vi "PhysioMoment.vi"() -> ()   [LabVIEW 2012]
doc: "Demonstrates general use of Obtain Queue, queues and the effects different settings have on queue behavior. It uses a queue to pass data between an Enqueue loop (producing data) and a Dequeue loop (consuming data). If both loops run at the same speed, the queue does not fill up.\n\nWhen the Enqueue loop runs fast and the Dequeue loop runs slow, the queue quickly fills up and the Enqueue loop must wait for the Dequeue loop to remove elements. If the Enqueue loop runs slow and the Dequeue loop runs fast, the queue is quickly emptied and the Dequeue loop must wait for the Enqueue loop to insert elements."
uses:
  <vilib>/Utility/file.llb/Read From Spreadsheet File (DBL).vi
  global_variable/tvi_arx_ni9234_global.vi
  <vilib>/Utility/file.llb/Read From Spreadsheet File (I64).vi
  <vilib>/Analysis/baseanly.llb/Mean (DBL).vi
  <vilib>/Analysis/NI_AALBase.lvlib
  <vilib>/Analysis/NI_AALPro.lvlib
panel:
  out "String":string="Ground Reaction Force \nBio-FeedBack System"
  out "output data size 2":i32
  out "transfer data size":i32
  out "transfer data":csg[](array[numeric])
  in  "Tab Control 2":enum32{"Settings", "Main Panel"}(tab)
  in  "Hours":i32
  in  "minutes":i32=14
  in  "seconds":i32
  in  "Loadcell Output Data":path
  in  "Led Runner File":path
  in  "Led Text File":path
  in  "Transfer Function":path
  out "Hours":i32
  out "minutes  2":i32=30
  out "seconds":i32
  in  "stop":bool
  in  "Tab Control":enum32{"GRF", "Raw Data"}(tab)
  out "10 SLOPE INCREMENT":dbl format="%#_3g"
  out "10 STRIDE INCREMENT":dbl format="%#_3g"
  out "5 SLOPE INCREMENT":dbl format="%#_3g"
  out "5 STRIDE INCREMENT":dbl format="%#_3g"
  out "1 SLOPE INCREMENT":dbl format="%#_3g"
  out "1 STRIDE INCREMENT":dbl format="%#_3g"
  out "TVItv SCORE":dbl format="%#_3g"
  out "Slope SCORE":dbl format="%#_3g"
  out "TVItv SCORE":dbl format="%#_3g"
  out "Slope SCORE":dbl format="%#_3g"
  out "Slope SCORE":dbl format="%#_3g"
  out "TVItv SCORE":dbl format="%#_3g"
  out "Bio-Feedback System":bool[][](array[boolean])
  out "Right Foot GRF":cluster{dbl[], "Z-Score":dbl[]}[](graph)
  out "Left Foot GRF":cluster{dbl[], "Z-Score":dbl[]}[](graph)
  out "TVItv Score : 1 stride":cluster{i32[], "Best Linear Fit":dbl[]}[](graph)
  out "TVItv Score : 5 strides":cluster{i32[], "Best Linear Fit":dbl[]}[](graph)
  out "TVItv Score : 10 strides":cluster{i32[], "Best Linear Fit":dbl[]}[](graph)
  out "GRF Output":dbl[](graph)
  out "GRF Input Waveform (2 Second Window)":cluster{dbl[], "Z-Score":dbl[]}[](graph)
  out "Step Interval (sec)":dbl
  out "tvit pr (1 strides)":dbl
  out "led loop execute time":dbl
  out "tvit (10 strides)":dbl
  out "tvit (10 strides)":dbl[](array[numeric])
  out "running phase":i8
  out "step-interval":dbl
  out "baseline value":dbl
  out "tvit array size\n(step count)":i32
  out "tvit (step)":dbl[](array[numeric])
  out "tvit (stride)":dbl
  out "tvit stride":dbl[](array[numeric])
  out "tvit stride array size":i32
  out "tvit (5 strides)":dbl[](array[numeric])
  out "tvit (5 strides)":dbl
  out "tvit pr (5 strides)":dbl
  out "mean":dbl
  out "new step interval":dbl
  out "new step global index":dbl
  out "Tvit of new step":dbl
  out "step-index":dbl[](array[numeric])
  out "step-length":dbl[](array[numeric])
  out "vaild Tvit":dbl[](array[numeric])
  out "points per loop":i32
  out "GRF Input size":i32
  out "GRF Output size":i32
  out "main loop":i32
  out "std(loadcell)":dbl
  out "new step index(global) in last loop":dbl
  out "window start index":i32
  out "new step interval in last loop":dbl
  out "counter (sec)":string
  out "loop execution time":dbl
  out "zero-crossing point\n(increasing)":dbl[](array[numeric])
  out "area between zero-crossing points \n(z-score series)":dbl[](array[numeric])
  out "interval between \nzero-crossing points":dbl[](array[numeric])
  out "zero-crossing interval\nlower threshold":dbl
  out "step-index\n(in window)":dbl[](array[numeric])
  # "Setting Time"
  # "Elapsed Time"
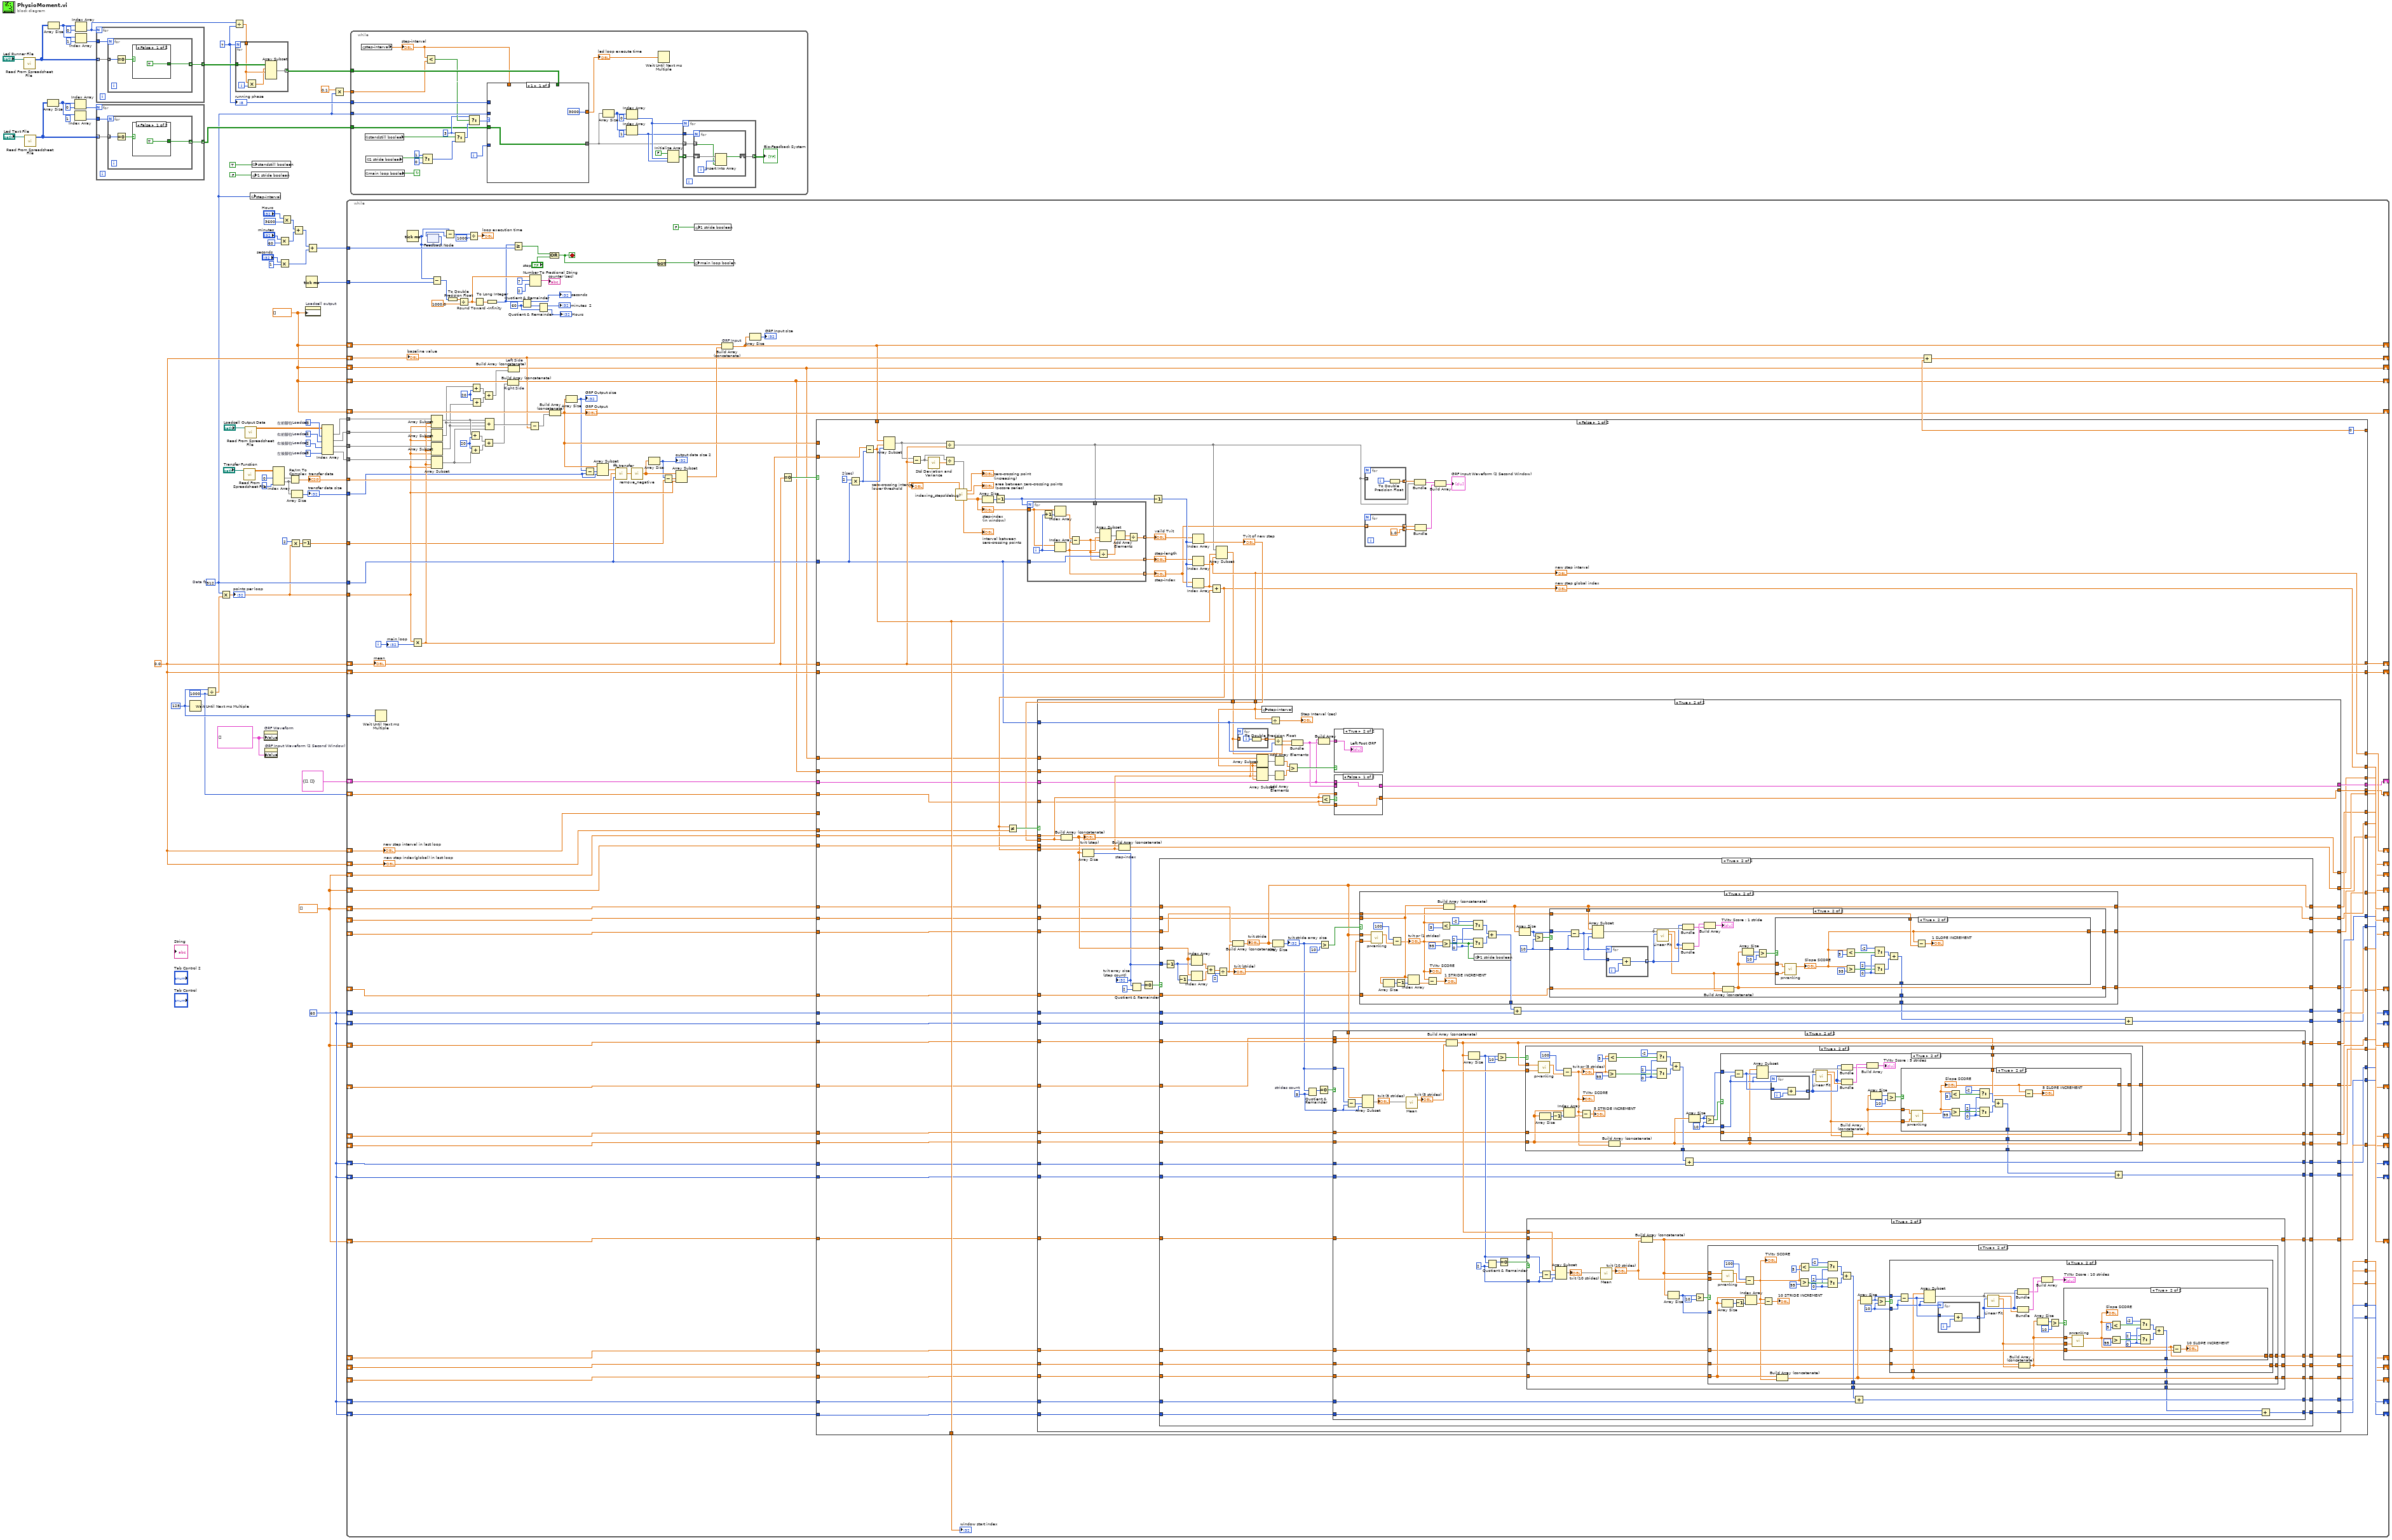
[diagram p0: block diagram]
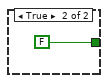
[diagram p2: hidden frame]
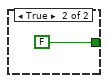
[diagram p3: hidden frame]
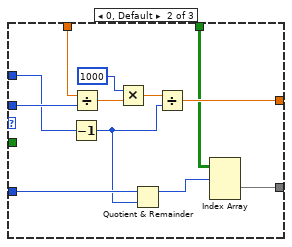
[diagram p4: hidden frame]
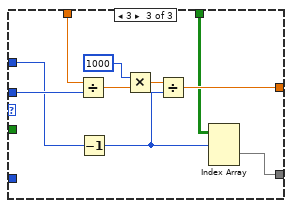
[diagram p5: hidden frame]
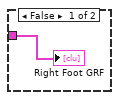
[diagram p8: hidden frame]
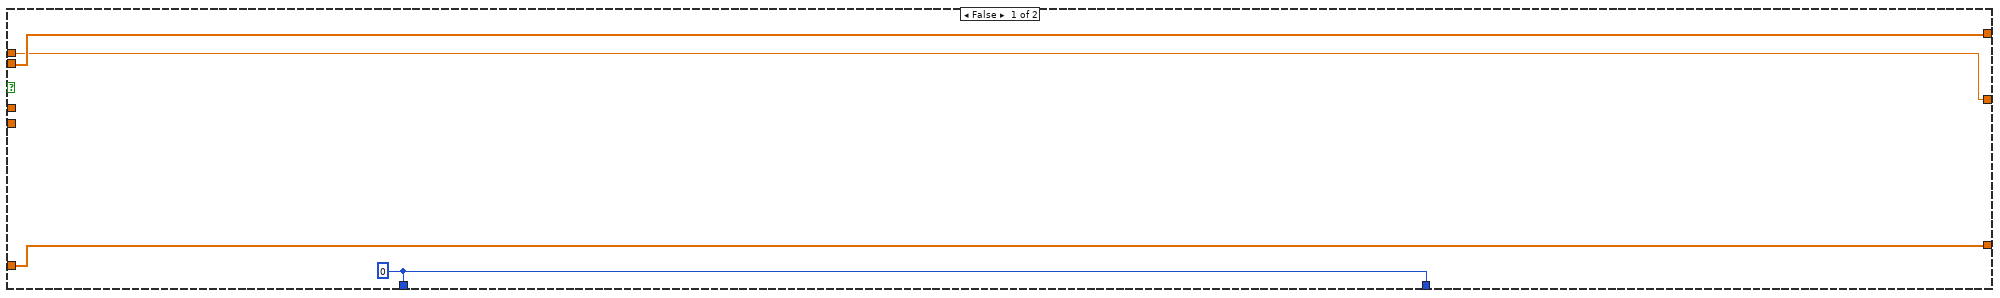
[diagram p10: hidden frame]
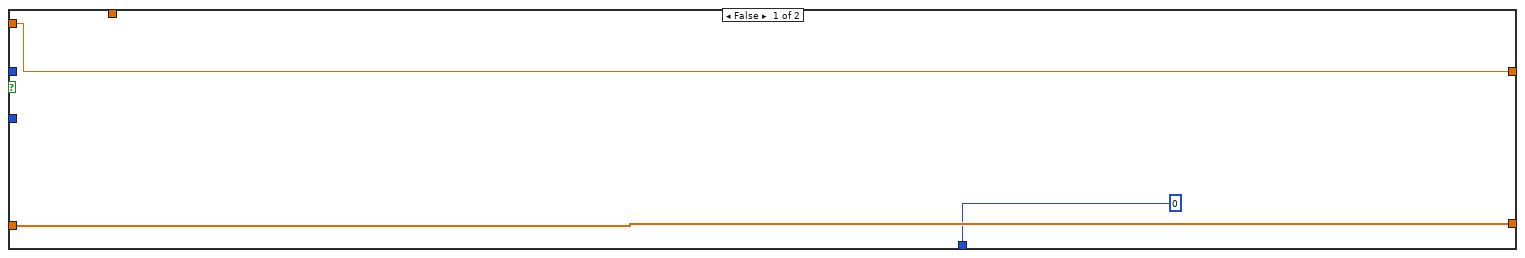
[diagram p11: hidden frame]
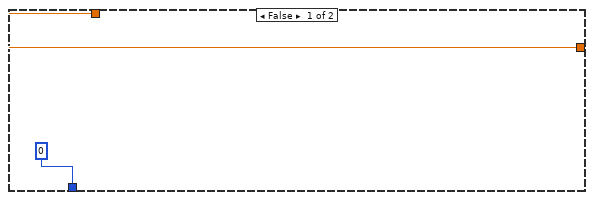
[diagram p12: hidden frame]
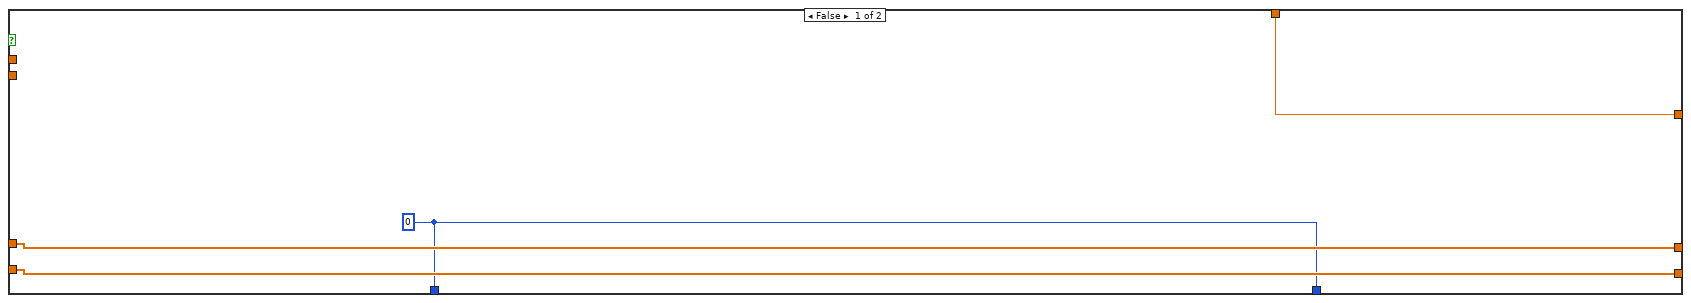
[diagram p14: hidden frame]
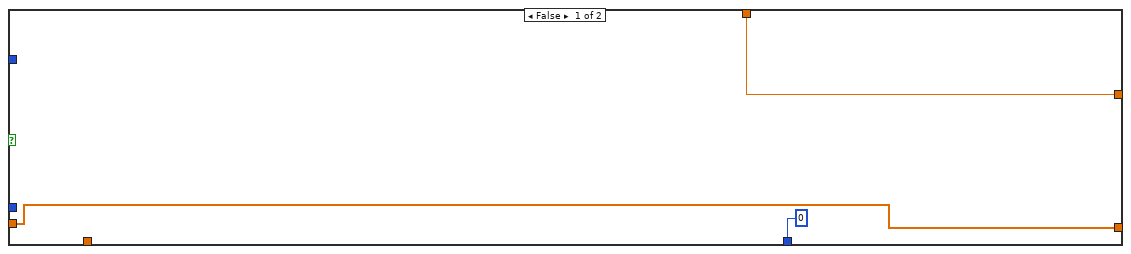
[diagram p15: hidden frame]
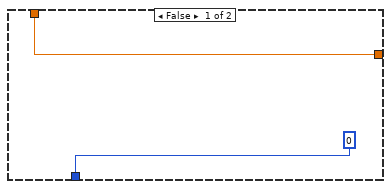
[diagram p16: hidden frame]
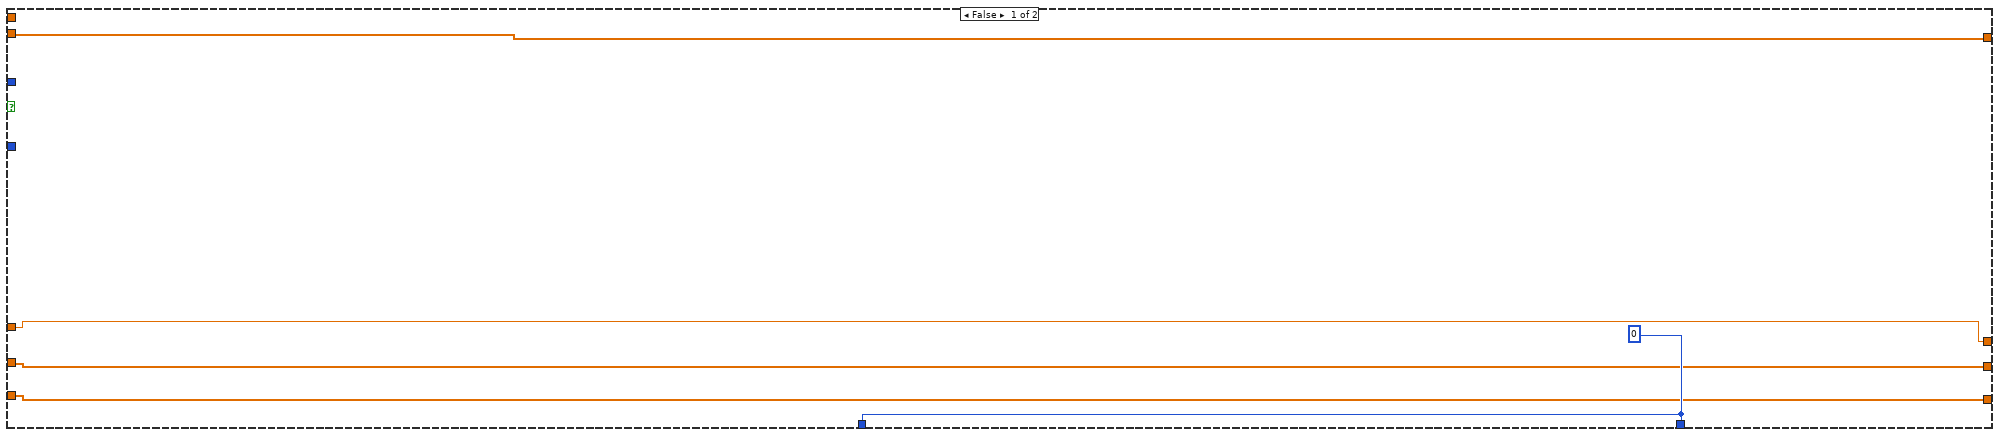
[diagram p17: hidden frame]
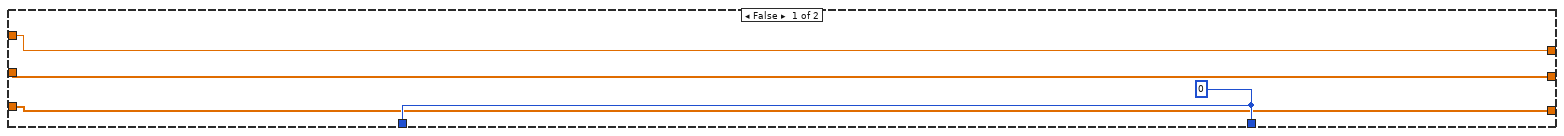
[diagram p18: hidden frame]
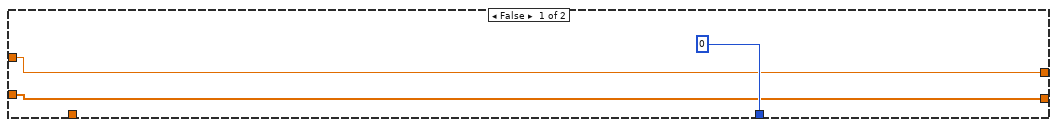
[diagram p19: hidden frame]
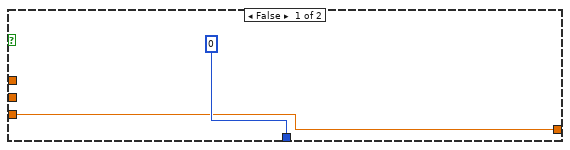
[diagram p20: hidden frame]
diagram:
  w24 = 60
  (unwired) 1
  w26 = 7
  w9 = dbl[] []
  w7 = cluster{dbl[], "Z-Score":dbl[]}[] [] ("Z-Score Waveform (2 sec)")
  w23 = 0.0
  w50 = 3  # 左後腳位Loadcell
  w51 = 2  # 右後腳位Loadcell
  w52 = 1  # 右前腳位Loadcell
  w53 = 0  # 左前腳位Loadcell
  w11 = 512  # Data fs
  w10 = dbl[] []
  w8 = 1000
  w48 = u32 125 ("millisecond multiple")
  n1 = call-poly <vilib>:"Read From Spreadsheet File.vi"("file path (dialog if empty)"="Led Runner File") -> ("all rows"=w37:i64[][])  [unwired: 6 in, 4 out]
  n2 = call-poly <vilib>:"Read From Spreadsheet File.vi"("file path (dialog if empty)"="Led Text File") -> ("all rows"=w31:i64[][])  [unwired: 6 in, 4 out]
  n3 = Array Size(array=w31) -> (size(s)=w32:i32[])
  n4 = Array Size(array=w37) -> (size(s)=w36:i32[])
  n5 = Index Array(array=w32, index=0) -> (element=w30:i32)
  n6 = Index Array(array=w32) -> (element=w29:i32)  [unwired: 1 in]
  n7 = Index Array(array=w36, index=0) -> (element=w27:i32)
  n8 = Index Array(array=w36, index=1) -> (element=w40:i32)
  n9 = for {
    N: w27 -> [_]
    tunnel: w37 -> [w69] mode=indexing
    tunnel: [w68] -> w39 mode=indexing
    tunnel: w40 -> [w67]
    n10 = for {
      N: w67 -> [_]
      tunnel: w69 -> [w71] mode=indexing
      tunnel: [w70] -> w68 mode=indexing
      n11 = Equal To 0?(x=w71) -> (x = 0?=w72:bool)
      n12 = case shown="False" w72 {
        tunnel: [TRUE FALSE] -> w70
        frame False {
        }
        frame True {
        }
      }
    }
  }
  n13 = for {
    N: w30 -> [_]
    tunnel: w31 -> [w77] mode=indexing
    tunnel: [w76] -> w28 mode=indexing
    tunnel: w29 -> [w75]
    n14 = for {
      N: w75 -> [_]
      tunnel: w77 -> [w79] mode=indexing
      tunnel: [w78] -> w76 mode=indexing
      n15 = Equal To 0?(x=w79) -> (x = 0?=w80:bool)
      n16 = case shown="False" w80 {
        tunnel: [TRUE FALSE] -> w78
        frame False {
        }
        frame True {
        }
      }
    }
  }
  n17 = Wait Until Next ms Multiple(millisecond multiple=w48) -> ()  [unwired: 1 out]
  n18 = Divide(x=w48, y=w8) -> (x/y=w47:dbl)
  n19 = Multiply(x=w11, y=w47) -> (x*y=w4:dbl)
  "points per loop" <- w4
  n20 = Divide(x=w27, y=w26) -> (x/y=w25:dbl)
  n21 = for {
    N: w26 -> [_]
    tunnel: w39 -> [w87]
    tunnel: w25 -> [w84]
    tunnel: [w85] -> w38 mode=indexing
    i -> [w86]
    n22 = Multiply(x=w84, y=w86) -> (x*y=w83:dbl)
    n23 = Array Subset(array=w87, index (row)=w83, length (row)=w84) -> (w85:bool[][])  [unwired: 2 in]
  }
  n24 = call-poly <vilib>:"Read From Spreadsheet File.vi"("file path (dialog if empty)"="Transfer Function") -> ("all rows"=w21:dbl[][])  [unwired: 6 in, 4 out]
  n25 = call-poly <vilib>:"Read From Spreadsheet File.vi"("file path (dialog if empty)"="Loadcell Output Data") -> ("all rows"=w49:dbl[][])  [unwired: 6 in, 4 out]
  n26 = global write "tvi_arx_ni9234_global.vi" "step-interval"(w11) -> ()
  n27 = global write "tvi_arx_ni9234_global.vi" "1 stride boolean"(FALSE) -> ()
  n28 = global write "tvi_arx_ni9234_global.vi" "standstill boolean"(TRUE) -> ()
  n29 = property on="GRF Waveform" class="XYGraph (strict)"("Value"=w7) -> ()  [unwired: 2 in, 2 out]
  n30 = property on="GRF Input Waveform (2 Second Window)" class="XYGraph (strict)"("Value"=w7) -> ()  [unwired: 2 in, 2 out]
  n31 = Index Array(array=w21, index (col) #1=0, index (col) #2=1) -> (element #1=w18:dbl[], element #2=w12:dbl[])  [unwired: 2 in]
  n32 = Multiply(x="minutes", y=60) -> (x*y=w65:i32)
  n33 = Multiply(x="seconds", y=1) -> (x*y=w56:i32)
  n34 = Multiply(x="Hours", y=3600) -> (x*y=w64:i32)
  n35 = Re/Im To Complex(1:w12, 2:w18) -> (0:w13:cdb[])
  "transfer data" <- w13
  n36 = Multiply(x=2, y=w4) -> (x*y=w2:dbl)
  n37 = Array Size(array=w12) -> (size(s)=w3:i32)
  "transfer data size" <- w3
  n38 = Add(x=w64, y=w65) -> (x+y=w57:i32)
  n39 = Decrement(x=w2) -> (x-1=w1:dbl)
  n40 = property on="Loadcell output" class="WFChart (strict)"("History Data"=w10) -> ()  [unwired: 2 in, 2 out]
  n41 = Tick Count (ms)() -> (millisecond timer value=w55:u32)
  n42 = Add(x=w57, y=w56) -> (x+y=w54:i32)
  n43 = Index Array(array=w49, index (col) #1=w53, index (col) #2=w52, index (col) #3=w51, index (col) #4=w50) -> (element #1=w17:dbl[], element #2=w16:dbl[], element #3=w15:dbl[], element #4=w14:dbl[])  [unwired: 4 in]
  n44 = Multiply(x=0.1, y=w11) -> (x*y=w34:dbl)
  n45 = while {
    tunnel: w55 -> [w206]
    tunnel: w54 -> [w205]
    tunnel: w48 -> [w202]
    shift-right: [w158] -> _
    shift-left: w23 -> [w173]
    shift-right: [w157] -> _
    shift-left: w23 -> [w172]
    tunnel: w4 -> [w109]
    shift-right: [w119] -> _
    shift-left: w10 -> [w189]
    tunnel: w11 -> [w118]
    shift-right: [w162] -> _
    shift-left: w10 -> [w188]
    shift-right: [w183] -> _
    shift-left: w23 -> [w184]
    shift-right: [w182] -> _
    shift-left: w23 -> [w181]
    shift-right: [w161] -> _
    shift-left: w9 -> [w179]
    shift-right: [w160] -> _
    shift-left: w9 -> [w178]
    shift-right: [w177] -> _
    shift-left: w9 -> [w176]
    shift-right: [w175] -> _
    shift-left: w9 -> [w174]
    tunnel: w17 -> [w171]
    tunnel: w16 -> [w170]
    tunnel: w15 -> [w169]
    tunnel: w14 -> [w168]
    shift-right: [w165] -> _
    shift-left: w23 -> [w163]
    shift-right: [w155] -> _
    shift-left: w9 -> [w154]
    shift-right: [w152] -> _
    shift-left: _ -> [w151]
    shift-right: [w150] -> _
    shift-left: w24 -> [w149]
    shift-right: [w148] -> _
    shift-left: w24 -> [w145]
    shift-right: [w147] -> _
    shift-left: _ -> [w146]
    shift-right: [w144] -> _
    shift-left: _ -> [w143]
    shift-right: [w142] -> _
    shift-left: w24 -> [w141]
    shift-right: [w138] -> _
    shift-left: w24 -> [w137]
    shift-right: [w140] -> _
    shift-left: _ -> [w139]
    shift-right: [w136] -> _
    shift-left: w24 -> [w130]
    shift-right: [w135] -> _
    shift-left: _ -> [w134]
    shift-right: [w133] -> _
    shift-left: _ -> [w132]
    shift-right: [w131] -> _
    shift-left: w24 -> [w129]
    shift-right: [w128] -> _
    shift-left: _ -> [w127]
    shift-right: [w126] -> _
    shift-left: _ -> [w125]
    shift-right: [w124] -> _
    shift-left: _ -> [w123]
    tunnel: w13 -> [w120]
    tunnel: w3 -> [w114]
    shift-right: [w94] -> _
    shift-left: w10 -> [w98]
    shift-right: [w93] -> _
    shift-left: w10 -> [w97]
    shift-right: [w89] -> _
    shift-left: cluster{dbl[], dbl[]} {[], []} -> [w92]
    shift-right: [w90] -> _
    shift-left: w8 -> [w91]
    tunnel: w1 -> [w88]
    i -> [w187]
    stop <- w159 stop-if-true
    w103 = 20
    w104 = 20
    w180 = 60 ("floor(x/y)")
    n46 = Wait Until Next ms Multiple(millisecond multiple=w202) -> ()  [unwired: 1 out]
    n47 = Tick Count (ms)() -> (millisecond timer value=w193:u32)
    n48 = Multiply(x=w109, y=w187) -> (x*y=w117:dbl)
    n49 = feedback-in #1(w193) -> ()
    n50 = feedback #1() -> (w198:u32)  [unwired: 1 in]
    n51 = Subtract(x=w193, y=w206) -> (x-y=w208:u32)
    n52 = Array Subset(array=w171, index=w117, length=w109) -> (w102:dbl[])
    n53 = Array Subset(array=w170, index=w117, length=w109) -> (w100:dbl[])
    n54 = Array Subset(array=w169, index=w117, length=w109) -> (w99:dbl[])
    n55 = Array Subset(array=w168, index=w117, length=w109) -> (w101:dbl[])
    n56 = Subtract(x=w193, y=w198) -> (x-y=w201:u32)
    n57 = To Double Precision Float(number=w208) -> (double precision float=w209:dbl)
    n58 = Divide(x=w209, y=1000.0) -> (x/y=w194:dbl)
    n59 = Divide(x=w201, y=1000) -> (x/y=→"loop execution time":dbl)
    n60 = Add(x=w102, y=w104) -> (x+y=w108:dbl[])
    n61 = Add(x=w104, y=w101) -> (x+y=w107:dbl[])
    n62 = Add(x=w100, y=w103) -> (x+y=w106:dbl[])
    n63 = Add(x=w103, y=w99) -> (x+y=w105:dbl[])
    n64 = Round Toward -Infinity(1:w194) -> (0:w207:dbl)
    n65 = Add(x=w106, y=w105) -> (x+y=w96:dbl[])
    n66 = Add(x=w108, y=w107) -> (x+y=w95:dbl[])
    n67 = Compound Arithmetic op=ADD(w102, w100, w99, w101) -> (w164:dbl[])
    n68 = To Long Integer(number=w207) -> (32bit integer=w191:i32)
    n69 = Build Array (concatenate) "Right Side"(w97, w95) -> (w93:dbl[])
    n70 = Build Array (concatenate) "Left Side"(w98, w96) -> (w94:dbl[])
    n71 = Greater Or Equal?(x=w191, y=w205) -> (x >= y?=w204:bool)
    n72 = Quotient & Remainder(x=w191, y=w180) -> (x-y*floor(x/y)=→"seconds":i32, floor(x/y)=w210:i32)
    n73 = Subtract(x=w164, y=w163) -> (x-y=w167:dbl[])
    n74 = Number To Fractional String(number=w194, width (-)=7, precision (6)=2) -> (F-format string=→"counter (sec)":string)  [unwired: 1 in]
    n75 = Quotient & Remainder(x=w210, y=w180) -> (x-y*floor(x/y)=→"minutes  2":i32, floor(x/y)=→"Hours":i32)
    n76 = Build Array (concatenate)(w189, w167) -> (w119:dbl[])
    "GRF Output" <- w119
    n77 = Compound Arithmetic op=OR(w204, "stop") -> (w159:bool)
    n78 = Array Size(array=w119) -> (size(s)=w115:i32)
    "GRF Output size" <- w115
    n79 = Subtract(x=w115, y=w114) -> (x-y=w116:i32)
    n80 = Array Subset(array=w119, index=w116, length=w114) -> (w122:dbl[])
    n81 = call "fft_transfer.vi"("Sample Rate"=w118, "Transfer Function"=w120, "GRF Output"=w122) -> ("GRF Input"=w121:dbl[])
    n82 = call "remove_negative.vi"("input array"=w121) -> ("output array"=w113:dbl[])
    n83 = Array Size(array=w113) -> (size(s)=w112:i32)
    "output data size 2" <- w112
    n84 = Not(x=w159) -> (.not. x?=w156:bool)
    n85 = Subtract(x=w112, y=w88) -> (x-y=w111:dbl)
    n86 = Array Subset(array=w113, index=w111, length=w109) -> (w110:dbl[])
    n87 = global write "tvi_arx_ni9234_global.vi" "main loop boolen"(w156) -> ()
    n88 = global write "tvi_arx_ni9234_global.vi" "1 stride boolean"(FALSE) -> ()
    n89 = Build Array (concatenate) "GRF Input"(w188, w110) -> (w162:dbl[])
    n90 = Array Size(array=w162) -> (size(s)=→"GRF Input size":i32)
    n91 = Equal To 0?(x=w181) -> (x = 0?=w190:bool)
    n92 = case shown="False" w190 {
      tunnel: w181 -> [w261 w822]
      tunnel: [w283 w805] -> w186
      tunnel: w118 -> [w251 w783]
      tunnel: w117 -> [w296 w803]
      tunnel: w119 -> [_ w811]
      tunnel: w184 -> [w272 w826]
      tunnel: [w272 w809] -> w183
      tunnel: [w252 w813] -> w158
      tunnel: [w256 w814] -> w157
      tunnel: [w261 w821] -> w182
      tunnel: w173 -> [w280 w813]
      tunnel: [w214 w818] -> w161
      tunnel: w179 -> [w279 w818]
      tunnel: [w278 w817] -> w160
      tunnel: w178 -> [w277 w817]
      tunnel: [w276 w816] -> w177
      tunnel: w176 -> [w275 w816]
      tunnel: [w274 w815] -> w175
      tunnel: w174 -> [w273 w815]
      tunnel: w172 -> [_ w814]
      tunnel: w162 -> [w270 w806]
      tunnel: [0 w804] -> w166
      tunnel: [w255 w802] -> w155
      tunnel: w154 -> [w254 w802]
      tunnel: [w250 w801] -> w152
      tunnel: w151 -> [w249 w801]
      tunnel: [w248 w799] -> w150
      tunnel: w149 -> [w247 w799]
      tunnel: [w246 w798] -> w148
      tunnel: [w245 w800] -> w147
      tunnel: w146 -> [w244 w800]
      tunnel: w145 -> [w243 w798]
      tunnel: [w242 w792] -> w144
      tunnel: w143 -> [w241 w792]
      tunnel: [w240 w791] -> w142
      tunnel: w141 -> [w239 w791]
      tunnel: [w238 w793] -> w140
      tunnel: w139 -> [w237 w793]
      tunnel: [w236 w790] -> w138
      tunnel: w137 -> [w235 w790]
      tunnel: [w234 w795] -> w136
      tunnel: [w233 w796] -> w135
      tunnel: w134 -> [w232 w796]
      tunnel: [w231 w797] -> w133
      tunnel: w132 -> [w230 w797]
      tunnel: [w229 w794] -> w131
      tunnel: w130 -> [w228 w795]
      tunnel: w129 -> [w227 w794]
      tunnel: [w226 w787] -> w128
      tunnel: w127 -> [w225 w787]
      tunnel: [w224 w788] -> w126
      tunnel: w125 -> [w223 w788]
      tunnel: [w222 w789] -> w124
      tunnel: w123 -> [w221 w789]
      tunnel: w94 -> [w220 _]
      tunnel: w93 -> [w219 _]
      tunnel: w92 -> [w218 w786]
      tunnel: w91 -> [w217 w785]
      tunnel: [w216 w785] -> w90
      tunnel: [w215 w786] -> w89
      frame False {
        w290 = 2  # 2(sec)
        n93 = Multiply(x=w290, y=w251) -> (x*y=w295:i32)
        n94 = Subtract(x=w296, y=w295) -> (x-y=w283:dbl)
        n95 = Array Subset(array=w270, index=w283, length=w295) -> (w258:dbl[])
        n96 = Subtract(x=w258, y=w261) -> (x-y=w259:dbl[])
        n97 = call <vilib>:"Std Deviation and Variance.vi"("X"=w259) -> ("standard deviation"=w297:dbl)  [unwired: 1 in, 2 out]
        n98 = Divide(x=w258, y=w261) -> (x/y=w257:dbl[])
        n99 = Divide(x=w259, y=w297) -> (x/y=w260:dbl[])
        n100 = call "indexing_steps(debug).vi"("z-score series (input)"=w260) -> ("lower threshold of zeros-interval"=→"zero-crossing interval\nlower threshold":dbl, "zeros-interval\n(interval between zero-crossing index)"=→"interval between \nzero-crossing points":dbl[], "increasing\nzero-crossing index"=→"zero-crossing point\n(increasing)":dbl[], "area between zero-crossing index"=→"area between zero-crossing points \n(z-score series)":dbl[], "index of steps (output)"=w288:dbl[])  [unwired: 1 in]
        "step-index\n(in window)" <- w288
        n101 = Array Size(array=w288) -> (size(s)=w289:i32)
        n102 = Decrement(x=w289) -> (x-1=w286:i32)
        n103 = for {
          N: w286 -> [_]
          tunnel: w288 -> [w775]
          tunnel: w257 -> [w778]
          tunnel: [w772] -> w285 mode=indexing
          tunnel: [w770] -> w284 mode=indexing
          tunnel: [w773] -> w263 mode=indexing
          tunnel: w251 -> [w774]
          i -> [w780]
          n104 = Increment(x=w780) -> (x+1=w781:i32)
          n105 = Index Array(array=w775, index=w781) -> (element=w779:dbl)
          n106 = Index Array(array=w775, index=w780) -> (element=w773:dbl)
          n107 = Subtract(x=w779, y=w773) -> (x-y=w770:dbl)
          n108 = Divide(x=w770, y=w774) -> (x/y=w771:dbl)
          n109 = Array Subset(array=w778, index=w773, length=w770) -> (w776:dbl[])
          n110 = Add Array Elements(numeric array=w776) -> (sum=w777:dbl)
          n111 = Divide(x=w777, y=w771) -> (x/y=w772:dbl)
        }
        "vaild Tvit" <- w285
        "step-length" <- w284
        "step-index" <- w263
        n112 = Decrement(x=w286) -> (x-1=w287:i32)
        n113 = Index Array(array=w285, index=w287) -> (element=w271:dbl)
        "Tvit of new step" <- w271
        n114 = Index Array(array=w284, index=w287) -> (element=w256:dbl)
        "new step interval" <- w256
        n115 = Index Array(array=w263, index=w287) -> (element=w282:dbl)
        n116 = Add(x=w282, y=w283) -> (x+y=w252:dbl)
        "new step global index" <- w252
        n117 = Not Equal?(x=w252, y=w280) -> (x != y?=w281:bool)
        n118 = Array Subset(array=w257, index=w282, length=w256) -> (w253:dbl[])
        n119 = case shown="True" w281 {
          tunnel: [w323 w377] -> w214
          tunnel: w279 -> [w323 w386]
          tunnel: w271 -> [_ w333]
          tunnel: [w321 w385] -> w278
          tunnel: w277 -> [w321 w384]
          tunnel: [w322 w383] -> w276
          tunnel: w275 -> [w322 w382]
          tunnel: [w320 w381] -> w274
          tunnel: w273 -> [w320 w380]
          tunnel: w256 -> [_ w329]
          tunnel: [w319 w379] -> w255
          tunnel: w254 -> [w319 w378]
          tunnel: w253 -> [_ w327]
          tunnel: w252 -> [_ w330]
          tunnel: w251 -> [_ w336]
          tunnel: [w318 w374] -> w250
          tunnel: w249 -> [w318 w373]
          tunnel: [w316 w372] -> w248
          tunnel: w247 -> [w316 w371]
          tunnel: [w315 w370] -> w246
          tunnel: [w317 w369] -> w245
          tunnel: w244 -> [w317 w368]
          tunnel: w243 -> [w315 w367]
          tunnel: [w313 w366] -> w242
          tunnel: w241 -> [w313 w365]
          tunnel: [w312 w364] -> w240
          tunnel: w239 -> [w312 w363]
          tunnel: [w314 w362] -> w238
          tunnel: w237 -> [w314 w361]
          tunnel: [w311 w360] -> w236
          tunnel: w235 -> [w311 w359]
          tunnel: [w308 w358] -> w234
          tunnel: [w309 w357] -> w233
          tunnel: w232 -> [w309 w356]
          tunnel: [w310 w355] -> w231
          tunnel: w230 -> [w310 w354]
          tunnel: [w307 w353] -> w229
          tunnel: w228 -> [w308 w352]
          tunnel: w227 -> [w307 w351]
          tunnel: [w304 w350] -> w226
          tunnel: w225 -> [w304 w349]
          tunnel: [w305 w348] -> w224
          tunnel: w223 -> [w305 w347]
          tunnel: [w306 w346] -> w222
          tunnel: w221 -> [w306 w345]
          tunnel: w220 -> [_ w339]
          tunnel: w219 -> [_ w338]
          tunnel: w218 -> [w303 w324]
          tunnel: w217 -> [w302 w332]
          tunnel: [w302 w334] -> w216
          tunnel: [w303 w326] -> w215
          frame False {
          }
          frame True {
            n120 = Build Array (concatenate)(w386, w333) -> (w377:dbl[])
            "tvit (step)" <- w377
            n121 = Array Size(array=w377) -> (size(s)=w376:i32)
            "tvit array size\n(step count)" <- w376
            n122 = Build Array (concatenate) "step-index"(w384, w330) -> (w385:dbl[])
            n123 = Quotient & Remainder(x=w376, y=2) -> (x-y*floor(x/y)=w389:i32)  [unwired: 1 out]
            n124 = Equal To 0?(x=w389) -> (x = 0?=w387:bool)
            n125 = case shown="True" w387 {
              tunnel: w377 -> [_ w465]
              tunnel: [w414 w450] -> w383
              tunnel: w376 -> [_ w464]
              tunnel: [w415 w457] -> w381
              tunnel: w382 -> [w414 w456]
              tunnel: w380 -> [w415 w455]
              tunnel: [w413 w454] -> w379
              tunnel: w378 -> [w413 w453]
              tunnel: [w412 w446] -> w374
              tunnel: w373 -> [w412 w447]
              tunnel: [w410 w443] -> w372
              tunnel: w371 -> [w410 w444]
              tunnel: [w409 w442] -> w370
              tunnel: [w411 w437] -> w369
              tunnel: w368 -> [w411 w438]
              tunnel: w367 -> [w409 w441]
              tunnel: [w407 w440] -> w366
              tunnel: w365 -> [w407 w439]
              tunnel: [w406 w435] -> w364
              tunnel: w363 -> [w406 w434]
              tunnel: [w408 w433] -> w362
              tunnel: w361 -> [w408 w432]
              tunnel: [w405 w431] -> w360
              tunnel: w359 -> [w405 w430]
              tunnel: [w402 w429] -> w358
              tunnel: [w403 w428] -> w357
              tunnel: w356 -> [w403 w427]
              tunnel: [w404 w426] -> w355
              tunnel: w354 -> [w404 w425]
              tunnel: [w401 w424] -> w353
              tunnel: w352 -> [w402 w423]
              tunnel: w351 -> [w401 w422]
              tunnel: [w398 w421] -> w350
              tunnel: w349 -> [w398 w420]
              tunnel: [w399 w419] -> w348
              tunnel: w347 -> [w399 w418]
              tunnel: [w400 w417] -> w346
              tunnel: w345 -> [w400 w416]
              frame False {
              }
              frame True {
                w466 = 5  # strides count
                n126 = Decrement(x=w464) -> (x-1=w462:i32)
                n127 = Decrement(x=w462) -> (x-1=w463:i32)
                n128 = Index Array(array=w465, index=w462) -> (element=w460:dbl)
                n129 = Index Array(array=w465, index=w463) -> (element=w461:dbl)
                n130 = Add(x=w460, y=w461) -> (x+y=w459:dbl)
                n131 = Divide(x=w459, y=2) -> (x/y=w451:dbl)
                "tvit (stride)" <- w451
                n132 = Build Array (concatenate)(w456, w451) -> (w450:dbl[])
                "tvit stride" <- w450
                n133 = Array Size(array=w450) -> (size(s)=w448:i32)
                "tvit stride array size" <- w448
                n134 = Quotient & Remainder(x=w448, y=w466) -> (x-y*floor(x/y)=w467:i32)  [unwired: 1 out]
                n135 = Equal To 0?(x=w467) -> (x = 0?=w468:bool)
                n136 = Greater?(x=w448, y=10) -> (0:w452:bool)
                n137 = case shown="True" w468 {
                  tunnel: w466 -> [_ w592]
                  tunnel: w450 -> [_ w594]
                  tunnel: w448 -> [_ w591]
                  tunnel: [w555 w585] -> w457
                  tunnel: w455 -> [w555 w589]
                  tunnel: [w554 w584] -> w454
                  tunnel: w453 -> [w554 w583]
                  tunnel: [w552 w579] -> w440
                  tunnel: w439 -> [w552 w578]
                  tunnel: [w551 w573] -> w435
                  tunnel: w434 -> [w551 w576]
                  tunnel: [w553 w575] -> w433
                  tunnel: w432 -> [w553 w574]
                  tunnel: [w550 w572] -> w431
                  tunnel: w430 -> [w550 w570]
                  tunnel: [w547 w566] -> w429
                  tunnel: [w548 w568] -> w428
                  tunnel: w427 -> [w548 w567]
                  tunnel: [w549 w565] -> w426
                  tunnel: w425 -> [w549 w564]
                  tunnel: [w546 w562] -> w424
                  tunnel: w423 -> [w547 w561]
                  tunnel: w422 -> [w546 w560]
                  tunnel: [w545 w559] -> w421
                  tunnel: w420 -> [w545 w558]
                  tunnel: [w544 w557] -> w419
                  tunnel: w418 -> [w544 w556]
                  frame False {
                  }
                  frame True {
                    w586 = 2
                    n138 = Subtract(x=w591, y=w592) -> (x-y=w593:i32)
                    n139 = Array Subset(array=w594, index=w593, length=w592) -> (w595:dbl[])
                    "tvit (5 strides)" <- w595
                    n140 = call-poly <vilib>:"Mean.vi"("X"=w595) -> ("mean"=w590:dbl)  [unwired: 1 out]
                    "tvit (5 strides)" <- w590
                    n141 = Build Array (concatenate)(w589, w590) -> (w585:dbl[])
                    n142 = Array Size(array=w585) -> (size(s)=w580:i32)
                    n143 = Quotient & Remainder(x=w580, y=w586) -> (x-y*floor(x/y)=w588:i32)  [unwired: 1 out]
                    n144 = Greater?(x=w580, y=10) -> (0:w582:bool)
                    n145 = Equal To 0?(x=w588) -> (x = 0?=w587:bool)
                    n146 = case shown="True" w582 {
                      tunnel: w590 -> [_ w628]
                      tunnel: w585 -> [_ w624]
                      tunnel: [w598 w609] -> w579
                      tunnel: w578 -> [w598 w604]
                      tunnel: [w597 w608] -> w577
                      tunnel: [w599 w607] -> w575
                      tunnel: w574 -> [w599 w606]
                      tunnel: [w597 w605] -> w571
                      tunnel: [w596 w603] -> w557
                      tunnel: w556 -> [w596 w602]
                      frame False {
                        w597 = 0
                      }
                      frame True {
                        w610 = 10
                        w619 = 0
                        n147 = call "pr-ranking.vi"("element"=w628, "Database Array"=w624) -> ("PR Value"=w620:dbl)  [unwired: 1 out]
                        n148 = Array Size(array=w604) -> (size(s)=w623:i32)
                        n149 = Decrement(x=w623) -> (x-1=w622:i32)
                        n150 = Subtract(x=100, y=w620) -> (x-y=w601:dbl)
                        "tvit pr (5 strides)" <- w601
                        "TVItv SCORE" <- w601
                        n151 = Index Array(array=w604, index=w622) -> (element=w621:dbl)
                        n152 = Subtract(x=w601, y=w621) -> (x-y=→"5 STRIDE INCREMENT":dbl)
                        n153 = Greater?(x=w601, y=95) -> (0:w613:bool)
                        n154 = Less?(x=w601, y=5) -> (x < y?=w614:bool)
                        n155 = Build Array (concatenate)(w604, w601) -> (w609:dbl[])
                        n156 = Select(t=-2, s=w614, f=w619) -> (s? t:f=w616:i32)
                        n157 = Select(t=2, s=w613, f=w619) -> (s? t:f=w615:i32)
                        n158 = Add(x=w616, y=w615) -> (x+y=w608:i32)
                        n159 = Array Size(array=w609) -> (size(s)=w611:i32)
                        n160 = Greater?(x=w611, y=w610) -> (0:w612:bool)
                        n161 = case shown="True" w612 {
                          tunnel: w611 -> [_ w644]
                          tunnel: w610 -> [_ w643]
                          tunnel: w609 -> [_ w642]
                          tunnel: [w630 w637] -> w607
                          tunnel: w606 -> [w630 w635]
                          tunnel: [0 w636] -> w605
                          tunnel: [w629 w634] -> w603
                          tunnel: w602 -> [w629 w633]
                          frame False {
                          }
                          frame True {
                            n162 = Subtract(x=w644, y=w643) -> (x-y=w650:i32)
                            n163 = Array Subset(array=w642, index=w650, length=w643) -> (w649:dbl[])
                            n164 = for {
                              N: w643 -> [_]
                              tunnel: w650 -> [w669]
                              tunnel: [w668] -> w641 mode=indexing
                              i -> [w670]
                              n165 = Add(x=w669, y=w670) -> (x+y=w668:i32)
                            }
                            n166 = call <vilib>:"Linear Fit.vi"("Y"=w649, "X"=w641) -> ("Best Linear Fit"=w648:dbl[], "slope"=w632:dbl)  [unwired: 9 in, 3 out]
                            n167 = Bundle(w641, w649) -> (w646:cluster{i32[], dbl[]})  [unwired: 1 in]
                            n168 = Bundle(w641, "Best Linear Fit"=w648) -> (w647:cluster{i32[], "Best Linear Fit":dbl[]})  [unwired: 1 in]
                            n169 = Build Array (concatenate)(w635, w632) -> (w637:dbl[])
                            n170 = Build Array(w647, w646) -> (→"TVItv Score : 5 strides":cluster{i32[], "Best Linear Fit":dbl[]}[])
                            n171 = Array Size(array=w637) -> (size(s)=w640:i32)
                            n172 = Greater?(x=w640, y=10) -> (0:w638:bool)
                            n173 = case shown="True" w638 {
                              tunnel: w637 -> [_ w667]
                              tunnel: w632 -> [_ w656]
                              tunnel: [0 w657] -> w636
                              tunnel: [w651 w654] -> w634
                              tunnel: w633 -> [w651 w655]
                              frame False {
                              }
                              frame True {
                                w664 = 0
                                n174 = call "pr-ranking.vi"("element"=w656, "Database Array"=w667) -> ("PR Value"=w654:dbl)  [unwired: 1 out]
                                "Slope SCORE" <- w654
                                n175 = Less?(x=w654, y=5) -> (x < y?=w659:bool)
                                n176 = Greater?(x=w654, y=95) -> (0:w658:bool)
                                n177 = Select(t=-2, s=w659, f=w664) -> (s? t:f=w661:i32)
                                n178 = Select(t=2, s=w658, f=w664) -> (s? t:f=w660:i32)
                                n179 = Add(x=w661, y=w660) -> (x+y=w657:i32)
                                n180 = Subtract(x=w654, y=w655) -> (x-y=→"5 SLOPE INCREMENT":dbl)
                              }
                            }
                          }
                        }
                      }
                    }
                    n181 = case shown="True" w587 {
                      tunnel: w586 -> [_ w691]
                      tunnel: w580 -> [_ w690]
                      tunnel: w585 -> [_ w689]
                      tunnel: [w675 w685] -> w584
                      tunnel: w583 -> [w675 w688]
                      tunnel: [w674 w683] -> w569
                      tunnel: [w673 w682] -> w568
                      tunnel: w567 -> [w673 w681]
                      tunnel: [w672 w680] -> w565
                      tunnel: w564 -> [w672 w679]
                      tunnel: [w674 w678] -> w563
                      tunnel: [w671 w677] -> w559
                      tunnel: w558 -> [w671 w676]
                      frame False {
                        w674 = 0
                      }
                      frame True {
                        n182 = Subtract(x=w690, y=w691) -> (x-y=w693:i32)
                        n183 = Array Subset(array=w689, index=w693, length=w691) -> (w694:dbl[])
                        "tvit (10 strides)" <- w694
                        n184 = call-poly <vilib>:"Mean.vi"("X"=w694) -> ("mean"=w692:dbl)  [unwired: 1 out]
                        "tvit (10 strides)" <- w692
                        n185 = Build Array (concatenate)(w688, w692) -> (w685:dbl[])
                        n186 = Array Size(array=w685) -> (size(s)=w684:i32)
                        n187 = Greater?(x=w684, y=10) -> (0:w686:bool)
                        n188 = case shown="True" w686 {
                          tunnel: w692 -> [_ w727]
                          tunnel: w685 -> [_ w720]
                          tunnel: w684 -> [_ _]
                          tunnel: [w698 w711] -> w683
                          tunnel: [w696 w707] -> w682
                          tunnel: w681 -> [w696 w703]
                          tunnel: [w697 w706] -> w680
                          tunnel: w679 -> [w697 w705]
                          tunnel: [w698 w704] -> w678
                          tunnel: [w695 w702] -> w677
                          tunnel: w676 -> [w695 w701]
                          frame False {
                            w698 = 0
                          }
                          frame True {
                            w709 = 10
                            w712 = 0
                            n189 = call "pr-ranking.vi"("element"=w727, "Database Array"=w720) -> ("PR Value"=w719:dbl)  [unwired: 1 out]
                            n190 = Array Size(array=w703) -> (size(s)=w723:i32)
                            n191 = Decrement(x=w723) -> (x-1=w722:i32)
                            n192 = Subtract(x=100, y=w719) -> (x-y=w700:dbl)
                            "TVItv SCORE" <- w700
                            n193 = Index Array(array=w703, index=w722) -> (element=w721:dbl)
                            n194 = Subtract(x=w700, y=w721) -> (x-y=→"10 STRIDE INCREMENT":dbl)
                            n195 = Build Array (concatenate)(w703, w700) -> (w707:dbl[])
                            n196 = Greater?(x=w700, y=95) -> (0:w713:bool)
                            n197 = Less?(x=w700, y=5) -> (x < y?=w714:bool)
                            n198 = Select(t=-2, s=w714, f=w712) -> (s? t:f=w716:i32)
                            n199 = Select(t=2, s=w713, f=w712) -> (s? t:f=w715:i32)
                            n200 = Add(x=w716, y=w715) -> (x+y=w711:i32)
                            n201 = Array Size(array=w707) -> (size(s)=w708:i32)
                            n202 = Greater?(x=w708, y=w709) -> (0:w710:bool)
                            n203 = case shown="True" w710 {
                              tunnel: w709 -> [_ w742]
                              tunnel: w708 -> [_ w741]
                              tunnel: w707 -> [_ w740]
                              tunnel: [w729 w736] -> w706
                              tunnel: w705 -> [w729 w734]
                              tunnel: [0 w735] -> w704
                              tunnel: [w728 w733] -> w702
                              tunnel: w701 -> [w728 w732]
                              frame False {
                              }
                              frame True {
                                n204 = Subtract(x=w741, y=w742) -> (x-y=w749:i32)
                                n205 = Array Subset(array=w740, index=w749, length=w742) -> (w746:dbl[])
                                n206 = for {
                                N: w742 -> [_]
                                tunnel: w749 -> [w768]
                                tunnel: [w767] -> w748 mode=indexing
                                i -> [w769]
                                n207 = Add(x=w768, y=w769) -> (x+y=w767:i32)
                                }
                                n208 = call <vilib>:"Linear Fit.vi"("Y"=w746, "X"=w748) -> ("Best Linear Fit"=w747:dbl[], "slope"=w731:dbl)  [unwired: 9 in, 3 out]
                                n209 = Bundle(w748, w746) -> (w744:cluster{i32[], dbl[]})  [unwired: 1 in]
                                n210 = Bundle(w748, "Best Linear Fit"=w747) -> (w745:cluster{i32[], "Best Linear Fit":dbl[]})  [unwired: 1 in]
                                n211 = Build Array (concatenate)(w734, w731) -> (w736:dbl[])
                                n212 = Array Size(array=w736) -> (size(s)=w739:i32)
                                n213 = Build Array(w745, w744) -> (→"TVItv Score : 10 strides":cluster{i32[], "Best Linear Fit":dbl[]}[])
                                n214 = Greater?(x=w739, y=10) -> (0:w737:bool)
                                n215 = case shown="True" w737 {
                                tunnel: w736 -> [_ w755]
                                tunnel: w731 -> [_ w756]
                                tunnel: [0 w757] -> w735
                                tunnel: [w750 w753] -> w733
                                tunnel: w732 -> [w750 w754]
                                frame False {
                                }
                                frame True {
                                w764 = 0
                                n216 = call "pr-ranking.vi"("element"=w756, "Database Array"=w755) -> ("PR Value"=w753:dbl)  [unwired: 1 out]
                                "Slope SCORE" <- w753
                                n217 = Less?(x=w753, y=5) -> (x < y?=w759:bool)
                                n218 = Greater?(x=w753, y=95) -> (0:w758:bool)
                                n219 = Select(t=-2, s=w759, f=w764) -> (s? t:f=w761:i32)
                                n220 = Select(t=2, s=w758, f=w764) -> (s? t:f=w760:i32)
                                n221 = Add(x=w761, y=w760) -> (x+y=w757:i32)
                                n222 = Subtract(x=w753, y=w754) -> (x-y=→"10 SLOPE INCREMENT":dbl)
                                }
                                }
                              }
                            }
                          }
                        }
                      }
                    }
                    n223 = Add(x=w577, y=w576) -> (x+y=w573:i32)
                    n224 = Add(x=w569, y=w561) -> (x+y=w566:i32)
                    n225 = Add(x=w571, y=w570) -> (x+y=w572:i32)
                    n226 = Add(x=w563, y=w560) -> (x+y=w562:i32)
                  }
                }
                n227 = case shown="True" w452 {
                  tunnel: w451 -> [_ w501]
                  tunnel: w450 -> [_ w497]
                  tunnel: [w472 w480] -> w446
                  tunnel: w447 -> [w472 w485]
                  tunnel: [w470 w488] -> w445
                  tunnel: w438 -> [w471 w479]
                  tunnel: [w471 w478] -> w437
                  tunnel: [w470 w477] -> w436
                  tunnel: [w469 w476] -> w417
                  tunnel: w416 -> [w469 w475]
                  frame False {
                    w470 = 0
                  }
                  frame True {
                    w482 = 10
                    w493 = 0
                    n228 = call "pr-ranking.vi"("element"=w501, "Database Array"=w497) -> ("PR Value"=w500:dbl)  [unwired: 1 out]
                    n229 = Array Size(array=w485) -> (size(s)=w487:i32)
                    n230 = Subtract(x=100, y=w500) -> (x-y=w473:dbl)
                    "tvit pr (1 strides)" <- w473
                    "TVItv SCORE" <- w473
                    n231 = Decrement(x=w487) -> (x-1=w486:i32)
                    n232 = Index Array(array=w485, index=w486) -> (element=w484:dbl)
                    n233 = Subtract(x=w473, y=w484) -> (x-y=→"1 STRIDE INCREMENT":dbl)
                    n234 = Less?(x=w473, y=5) -> (x < y?=w495:bool)
                    n235 = Greater?(x=w473, y=95) -> (0:w494:bool)
                    n236 = Build Array (concatenate)(w485, w473) -> (w480:dbl[])
                    n237 = Select(t=-2, s=w495, f=w493) -> (s? t:f=w490:i32)
                    n238 = Select(t=2, s=w494, f=w493) -> (s? t:f=w489:i32)
                    n239 = global write "tvi_arx_ni9234_global.vi" "1 stride boolean"(w494) -> ()
                    n240 = Add(x=w490, y=w489) -> (x+y=w488:i32)
                    n241 = Array Size(array=w480) -> (size(s)=w483:i32)
                    n242 = Greater?(x=w483, y=w482) -> (0:w481:bool)
                    n243 = case shown="True" w481 {
                      tunnel: w482 -> [_ w516]
                      tunnel: w483 -> [_ w515]
                      tunnel: w480 -> [_ w514]
                      tunnel: [w504 w509] -> w478
                      tunnel: w479 -> [w504 w513]
                      tunnel: [0 w508] -> w477
                      tunnel: [w502 w506] -> w476
                      tunnel: w475 -> [w502 w505]
                      frame False {
                      }
                      frame True {
                        n244 = Subtract(x=w515, y=w516) -> (x-y=w517:i32)
                        n245 = Array Subset(array=w514, index=w517, length=w516) -> (w520:dbl[])
                        n246 = for {
                          N: w516 -> [_]
                          tunnel: w517 -> [w542]
                          tunnel: [w541] -> w519 mode=indexing
                          i -> [w543]
                          n247 = Add(x=w542, y=w543) -> (x+y=w541:i32)
                        }
                        n248 = call <vilib>:"Linear Fit.vi"("Y"=w520, "X"=w519) -> ("Best Linear Fit"=w518:dbl[], "slope"=w507:dbl)  [unwired: 9 in, 3 out]
                        n249 = Bundle(w519, w520) -> (w521:cluster{i32[], dbl[]})  [unwired: 1 in]
                        n250 = Bundle(w519, "Best Linear Fit"=w518) -> (w522:cluster{i32[], "Best Linear Fit":dbl[]})  [unwired: 1 in]
                        n251 = Build Array(w522, w521) -> (→"TVItv Score : 1 stride":cluster{i32[], "Best Linear Fit":dbl[]}[])
                        n252 = Build Array (concatenate)(w513, w507) -> (w509:dbl[])
                        n253 = Array Size(array=w509) -> (size(s)=w512:i32)
                        n254 = Greater?(x=w512, y=10) -> (0:w510:bool)
                        n255 = case shown="True" w510 {
                          tunnel: w509 -> [_ w540]
                          tunnel: w507 -> [_ w529]
                          tunnel: [0 w530] -> w508
                          tunnel: [w524 w527] -> w506
                          tunnel: w505 -> [w524 w528]
                          frame False {
                          }
                          frame True {
                            w537 = 0
                            n256 = call "pr-ranking.vi"("element"=w529, "Database Array"=w540) -> ("PR Value"=w527:dbl)  [unwired: 1 out]
                            "Slope SCORE" <- w527
                            n257 = Less?(x=w527, y=5) -> (x < y?=w532:bool)
                            n258 = Greater?(x=w527, y=95) -> (0:w531:bool)
                            n259 = Select(t=-2, s=w532, f=w537) -> (s? t:f=w534:i32)
                            n260 = Select(t=2, s=w531, f=w537) -> (s? t:f=w533:i32)
                            n261 = Add(x=w534, y=w533) -> (x+y=w530:i32)
                            n262 = Subtract(x=w527, y=w528) -> (x-y=→"1 SLOPE INCREMENT":dbl)
                          }
                        }
                      }
                    }
                  }
                }
                n263 = Add(x=w445, y=w444) -> (x+y=w443:i32)
                n264 = Add(x=w436, y=w441) -> (x+y=w442:i32)
              }
            }
            n265 = for {
              tunnel: [w394] -> w337 mode=indexing
              tunnel: w327 -> [_] mode=indexing
              i -> [w395]
              n266 = To Double Precision Float(number=w395) -> (double precision float=w394:dbl)
            }
            n267 = Array Subset(array=w339, index=w330, length=w329) -> (w344:dbl[])
            n268 = Array Subset(array=w338, index=w330, length=w329) -> (w343:dbl[])
            n269 = global write "tvi_arx_ni9234_global.vi" "step-interval"(w329) -> ()
            n270 = Divide(x=w329, y=w336) -> (x/y=→"Step Interval (sec)":dbl)
            n271 = Divide(x=w337, y=w336) -> (x/y=w328:dbl[])
            n272 = Add Array Elements(numeric array=w344) -> (sum=w341:dbl)
            n273 = Add Array Elements(numeric array=w343) -> (sum=w342:dbl)
            n274 = Greater?(x=w341, y=w342) -> (0:w340:bool)
            n275 = Bundle(w328, w327) -> (w325:cluster{dbl[], dbl[]})  [unwired: 1 in]
            n276 = Build Array(w324, w325) -> (w331:cluster{dbl[], dbl[]}[])
            n277 = Less?(x=w333, y=w332) -> (x < y?=w335:bool)
            n278 = case shown="True" w340 {
              tunnel: w331 -> [w396 w397]
              frame False {
                "Right Foot GRF" <- w396
              }
              frame True {
                "Left Foot GRF" <- w397
              }
            }
            n279 = case shown="False" w335 {
              tunnel: [w391 w393] -> w334
              tunnel: w333 -> [_ w393]
              tunnel: w332 -> [w391 _]
              tunnel: [w390 w392] -> w326
              tunnel: w324 -> [w390 _]
              tunnel: w325 -> [_ w392]
              frame False {
              }
              frame True {
              }
            }
          }
        }
        n280 = for {
          tunnel: [w298] -> w264 mode=indexing
          tunnel: w257 -> [_] mode=indexing
          i -> [w299]
          n281 = To Double Precision Float(number=w299) -> (double precision float=w298:dbl)
        }
        n282 = for {
          tunnel: [w301] -> w269 mode=indexing
          tunnel: w263 -> [w301] mode=indexing
          tunnel: [1.0] -> w268 mode=indexing
        }
        n283 = Bundle(w264, w257) -> (w266:cluster{dbl[], dbl[]})  [unwired: 1 in]
        n284 = Bundle(w269, w268) -> (w267:cluster{dbl[], dbl[]})  [unwired: 1 in]
        n285 = Build Array(w266, w267) -> (→"GRF Input Waveform (2 Second Window)":cluster{dbl[], dbl[]}[])
      }
      frame True {
        w782 = 2  # 2(sec)
        n286 = Multiply(x=w783, y=w782) -> (x*y=w819:i32)
        n287 = Divide(x=w783, y=w782) -> (x/y=w784:dbl)
        n288 = Subtract(x=w803, y=w819) -> (x-y=w805:dbl)
        n289 = Array Subset(array=w811, index=w805, length=w819) -> (w820:dbl[])
        n290 = call <vilib>:"Std Deviation and Variance.vi"("X"=w820) -> ("standard deviation"=w823:dbl)  [unwired: 1 in, 2 out]
        "std(loadcell)" <- w823
        n291 = Greater?(x=w823, y=0.9999999999999997 ("標準差門檻值")) -> (0:w812:bool)
        n292 = case shown="True" w812 {
          tunnel: w826 -> [w872 w877]
          tunnel: [w873 w876] -> w809
          tunnel: w784 -> [_ w874]
          frame False {
            n293 = Multiply(x=0, y=w872) -> (x*y=w873:dbl)
          }
          frame True {
            n294 = Increment(x=w877) -> (x+1=w876:dbl)
            n295 = global write "tvi_arx_ni9234_global.vi" "standstill boolean"(FALSE) -> ()
            n296 = global write "tvi_arx_ni9234_global.vi" "step-interval"(w874) -> ()
          }
        }
        n297 = Equal?(x=w809, y=64) -> (x = y?=w824:bool)
        n298 = Equal?(x=w809, y=144) -> (x = y?=w808:bool)
        n299 = case shown="True" w808 {
          tunnel: [0 w833] -> w807
          tunnel: w783 -> [_ w841]
          tunnel: w806 -> [_ w832]
          tunnel: w803 -> [_ w842]
          frame False {
          }
          frame True {
            w843 = 8  # 8(sec)
            n300 = Multiply(x=w843, y=w841) -> (x*y=w845:i32)
            n301 = Subtract(x=w842, y=w845) -> (x-y=w844:dbl)
            n302 = Array Subset(array=w832, index=w844, length=w845) -> (w829:dbl[])
            n303 = call "z-score.vi"("Array"=w829) -> ("Z-Score"=w831:dbl[])  [unwired: 2 out]
            n304 = call "indexing_steps.vi"("z-score series (input)"=w831) -> ("index of step (output)"=w830:dbl[])  [unwired: 5 in]
            n305 = Array Size(array=w830) -> (size(s)=w836:i32)
            n306 = Decrement(x=w836) -> (x-1=w834:i32)
            n307 = Index Array(array=w830, index=w834) -> (element=w840:dbl)
            n308 = Index Array(array=w830, index=0) -> (element=w839:dbl)
            n309 = Subtract(x=w840, y=w839) -> (x-y=w838:dbl)
            n310 = Array Subset(array=w829, index=w839, length=w838) -> (w837:dbl[])
            n311 = call-poly <vilib>:"Mean.vi"("X"=w837) -> ("mean"=w833:dbl)  [unwired: 1 out]
          }
        }
        n312 = case shown="True" w824 {
          tunnel: w811 -> [_ w856]
          tunnel: w803 -> [_ w854]
          tunnel: w783 -> [_ w852]
          tunnel: [0 w848] -> w804
          frame False {
          }
          frame True {
            w855 = 8  # 8(sec)
            n313 = Multiply(x=w855, y=w852) -> (x*y=w851:i32)
            n314 = Subtract(x=w854, y=w851) -> (x-y=w853:dbl)
            n315 = Array Subset(array=w856, index=w853, length=w851) -> (w847:dbl[])
            n316 = Sort 1D Array(array=w847) -> (sorted array=w850:dbl[])
            n317 = while {
              tunnel: w850 -> [w857]
              tunnel: 8 -> [w859]
              tunnel: [w863] -> w848
              i -> [w862]
              stop <- w869 stop-if-true
              n318 = Increment(x=w862) -> (x+1=w860:i32)
              n319 = Multiply(x=w860, y=w859) -> (x*y=w858:i32)
              n320 = Multiply(x=w859, y=w862) -> (x*y=w861:i32)
              n321 = Array Subset(array=w857, index=w858, length=w859) -> (w868:dbl[])
              n322 = Array Subset(array=w857, index=w861, length=w859) -> (w867:dbl[])
              n323 = call-poly <vilib>:"Mean.vi"("X"=w867) -> ("mean"=w865:dbl)  [unwired: 1 out]
              n324 = call-poly <vilib>:"Mean.vi"("X"=w868) -> ("mean"=w866:dbl)  [unwired: 1 out]
              n325 = Subtract(x=w866, y=w865) -> (x-y=w864:dbl)
              n326 = Greater?(x=w864, y=-5e-05) -> (0:w869:bool)
              n327 = Index Array(array=w857, index=w858) -> (element=w863:dbl)
            }
          }
        }
        n328 = Add(x=w807, y=w822) -> (x+y=w821:dbl)
      }
    }
    "window start index" <- w186
    n329 = Add(x=w163, y=w166) -> (x+y=w165:dbl)
    "new step interval in last loop" <- w172
    "new step index(global) in last loop" <- w173
    "main loop" <- w187
    "mean" <- w181
    "baseline value" <- w163
  }
  n330 = while {
    tunnel: w38 -> [w899]
    tunnel: w11 -> [w897]
    tunnel: w26 -> [w900]
    tunnel: w34 -> [w884]
    tunnel: w28 -> [w879]
    i -> [w901]
    stop <- w904 continue-if-true
    w881 = 3
    n331 = global read "tvi_arx_ni9234_global.vi" "step-interval"() -> (w885:dbl)
    "step-interval" <- w885
    n332 = global read "tvi_arx_ni9234_global.vi" "standstill boolean"() -> (w895:bool)
    n333 = global read "tvi_arx_ni9234_global.vi" "main loop boolen"() -> (w904:bool)
    n334 = global read "tvi_arx_ni9234_global.vi" "1 stride boolean"() -> (w898:bool)
    n335 = Select(t=1, s=w898, f=0) -> (s? t:f=w878:i32)
    n336 = Less?(x=w885, y=w884) -> (x < y?=w883:bool)
    n337 = Select(t=w881, s=w895, f=w878) -> (s? t:f=w880:i32)
    n338 = Select(t=w881, s=w883, f=w880) -> (s? t:f=w882:i32)
    n339 = case shown="1" w882 {
      tunnel: w901 -> [_ w926 _]
      tunnel: w900 -> [_ w919 w930]
      tunnel: w899 -> [_ w917 w928]
      tunnel: w897 -> [_ w922 w932]
      tunnel: w885 -> [_ w921 w933]
      tunnel: [3000 w920 w931] -> w896
      tunnel: [w913 w915 w929] -> w886
      tunnel: w879 -> [w913 _ _]
      frame 1 {
      }
      frame 0, Default {
        n340 = Decrement(x=w919) -> (x-1=w918:i32)
        n341 = Divide(x=w921, y=w922) -> (x/y=w924:dbl)
        n342 = Multiply(x=1000, y=w924) -> (x*y=w925:dbl)
        n343 = Quotient & Remainder(x=w926, y=w918) -> (x-y*floor(x/y)=w916:i32)  [unwired: 1 out]
        n344 = Divide(x=w925, y=w918) -> (x/y=w920:dbl)
        n345 = Index Array(array=w917, index (dim 0)=w916) -> (element=w915:bool[][])  [unwired: 2 in]
      }
      frame 3 {
        n346 = Divide(x=w933, y=w932) -> (x/y=w935:dbl)
        n347 = Decrement(x=w930) -> (x-1=w927:i32)
        n348 = Multiply(x=1000, y=w935) -> (x*y=w936:dbl)
        n349 = Divide(x=w936, y=w927) -> (x/y=w931:dbl)
        n350 = Index Array(array=w928, index (dim 0)=w927) -> (element=w929:bool[][])  [unwired: 2 in]
      }
    }
    "led loop execute time" <- w896
    n351 = Array Size(array=w886) -> (size(s)=w889:i32[])
    n352 = Index Array(array=w889, index=0) -> (element=w888:i32)
    n353 = Index Array(array=w889, index=1) -> (element=w887:i32)
    n354 = Wait Until Next ms Multiple(millisecond multiple=w896) -> ()  [unwired: 1 out]
    n355 = Initialize Array(FALSE, w888, w887) -> (w893:bool[][])
    n356 = for {
      N: w888 -> [_]
      tunnel: [w908] -> w890 mode=indexing
      tunnel: w886 -> [w907] mode=indexing
      tunnel: w893 -> [w906] mode=indexing
      tunnel: w887 -> [w905]
      n357 = for {
        N: w905 -> [_]
        tunnel: w907 -> [w909] mode=indexing
        shift-right: [w912] -> w908
        shift-left: w906 -> [w910]
        i -> [w911]
        n358 = Insert Into Array(array=w910, index=w911, new element=w909) -> (w912:bool[])
      }
    }
    "Bio-Feedback System" <- w890
  }
  "running phase" <- w26
